vi "Polling Start Core.vi"(8 "Error In":errorcluster, 11 "CS++BaseActor in":refnum<class "CS++BaseActor.lvclass">) -> (0 "Error Out":errorcluster, 3 "CS++BaseActor out":refnum<class "CS++BaseActor.lvclass">)   [LabVIEW 2016, in "CS++BaseActor.lvlib" / "CS++BaseActor.lvclass"]
doc: "Implement your code to start polling here."
uses:
  CS++BaseActor.lvclass
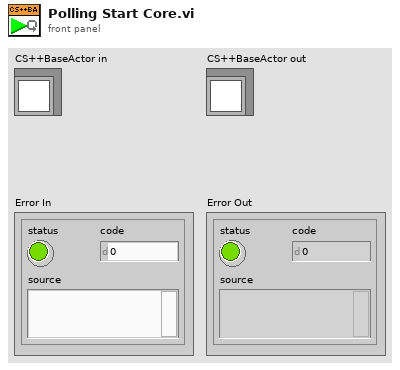
[diagram p1: front panel]
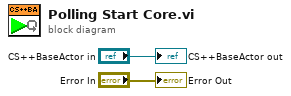
[diagram p0: block diagram]
diagram:
  "Error Out" <- "Error In"
  "CS++BaseActor out" <- "CS++BaseActor in"
